vi "Instrument Mode.vi"(4 "SKIP(T)":bool, 6 "SET/GET":string(combo)="SET", 8 "error in":errorcluster {"code" format="%.0x"}, 9 "Select INST":string(combo)="INST SA", 11 "Session In":refnum<visa-resource-name>="TCPIP0::169.254.70.120::inst0::INSTR") -> (0 "error out":errorcluster={"status"=TRUE, "code"=-1073807339, "source"="VISA Write in Instrument Mode.vi"} {"code" format="%.0x"}, 2 "INST":string="INST SA", 3 "Session Out":refnum<visa-resource-name>="TCPIP0::169.254.70.120::inst0::INSTR")   [LabVIEW 2018]
doc: "Launches the Instrument I/O Assistant, which you can use to communicate with message-based instruments and graphically parse the response. For example you can communicate with an instrument that uses a serial, Ethernet, or GPIB interface."
panel:
  # ":INSTrument[:SELect] SA | RTSA | SEQAN | EMI | BASIC | WCDMA |\nEDGEGSM | WIMAXOFDMA | VSA | PNOISE | NFIGure | ADEMOD | BTooth |\nTDSCDMA | CDMA2K | CDMA1XEV | LTE | LTETDD | LTEAFDD | LTEATDD | MSR\n| DVB | DTMB | DCTV | ISDBT | CMMB | WLAN | CWLAN | CWIMAXOFDM |\nWIMAXFIXED | IDEN | RLC | SCPILC | VSA89601\n:INSTrument[:SELect]?"
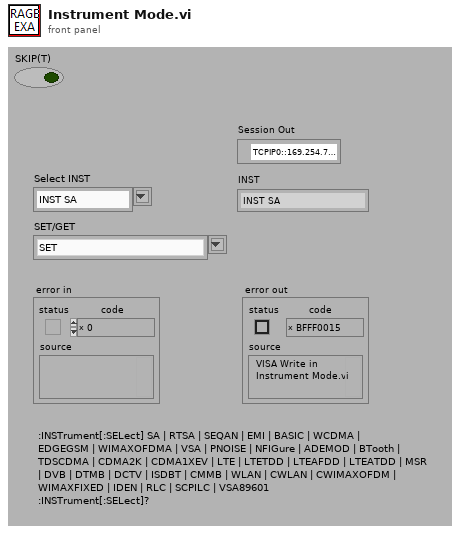
[diagram p1: front panel]
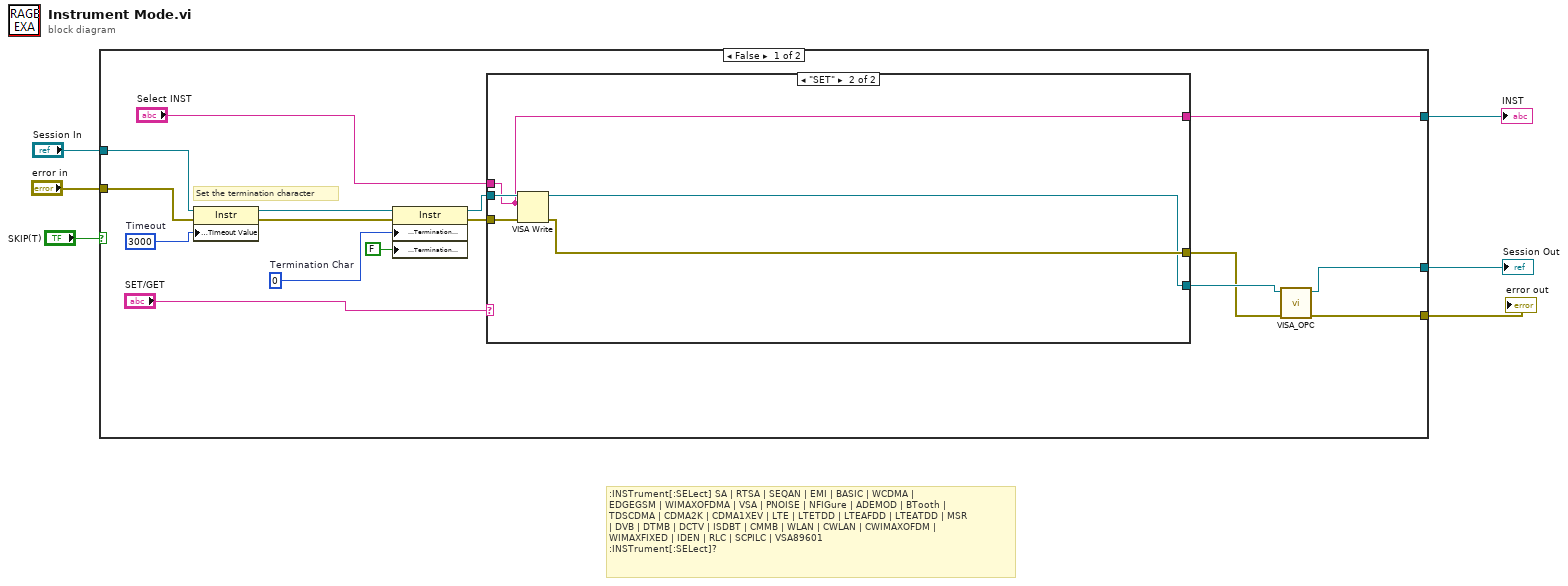
[diagram p0: block diagram]
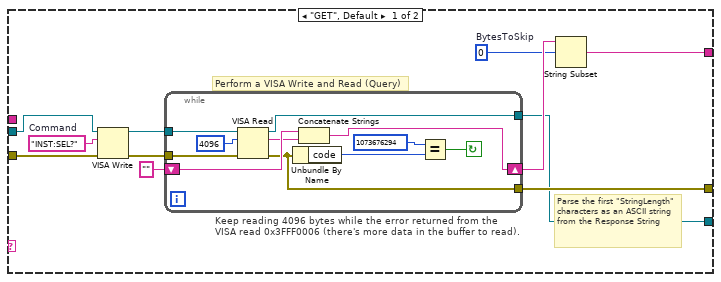
[diagram p2: hidden frame]
diagram:
  # ":INSTrument[:SELect] SA | RTSA | SEQAN | EMI | BASIC | WCDMA |\nEDGEGSM | WIMAXOFDMA | VSA | PNOISE | NFIGure | ADEMOD | BTooth |\nTDSCDMA | CDMA2K | CDMA1XEV | LTE | LTETDD | LTEAFDD | LTEATDD | MSR\n| DVB | DTMB | DCTV | ISDBT | CMMB | WLAN | CWLAN | CWIMAXOFDM |\nWIMAXFIXED | IDEN | RLC | SCPILC | VSA89601\n:INSTrument[:SELect]?"
  n1 = case shown="False" "SKIP(T)" {
    tunnel: "error in" -> [w21 w51]
    tunnel: "Session In" -> [w20 w50]
    tunnel: [w14 w50] -> w4
    tunnel: [w10 w50] -> w3
    tunnel: [w8 w51] -> w2
    frame False {
      w17 = u8 0  # Termination Char
      w22 = u32 3000  # Timeout
      # "Set the termination character"
      n2 = property class="Instr"(reference=w20, error in=w21, "General Settings:Timeout Value"=w22) -> (reference out=w16:refnum<visa-resource-name>, error out=w19:errorcluster)
      n3 = property class="Instr"(reference=w16, error in=w19, "Message Based Settings:Termination Character"=w17, "Message Based Settings:Termination Character Enable"=FALSE ("enable")) -> (reference out=w12:refnum<visa-resource-name>, error out=w18:errorcluster)
      n4 = case shown="\"SET\"" "SET/GET" {
        tunnel: w18 -> [w33 w49]
        tunnel: [w30 w48] -> w7
        tunnel: [w27 w45] -> w14
        tunnel: w12 -> [w24 w47]
        tunnel: "Select INST" -> [_ w45]
        tunnel: [w23 w46] -> w9
        frame "GET", Default {
          w25 = 0  # BytesToSkip
          w28 = "INST:SEL?"  # Command
          # "Parse the first \"StringLength\" characters as an ASCII string from the Response String"
          # "Perform a VISA Write and Read (Query)"
          # "Keep reading 4096 bytes while the error returned from the\nVISA read 0x3FFF0006 (there's more data in the buffer to read)."
          n5 = VISA Write(VISA resource name=w24, write buffer=w28, error in (no error)=w33) -> (VISA resource name out=w32:refnum<visa-resource-name>, error out=w31:errorcluster)  [unwired: 1 out]
          n6 = while {
            tunnel: w32 -> [w41]
            shift-right: [w35] -> w26
            shift-left: "" -> [w40]
            tunnel: w31 -> [w38]
            tunnel: [w37] -> w30
            tunnel: [w34] -> w23
            stop <- w36 continue-if-true
            n7 = VISA Read(VISA resource name=w41, byte count=u32 4096 ("byte count (0)"), error in (no error)=w38) -> (VISA resource name out=w34:refnum<visa-resource-name>, read buffer=w39:string, error out=w37:errorcluster)  [unwired: 1 out]
            n8 = Unbundle By Name(w37) -> ("code"=w43:i32)
            n9 = Concatenate Strings(w40, w39) -> (w35:string)
            n10 = Equal?(x=1073676294, y=w43) -> (x = y?=w36:bool)
          }
          n11 = String Subset(string=w26, offset (0)=w25) -> (substring=w27:string)  [unwired: 1 out]
        }
        frame "SET" {
          n12 = VISA Write(VISA resource name=w47, write buffer=w45, error in (no error)=w49) -> (VISA resource name out=w46:refnum<visa-resource-name>, error out=w48:errorcluster)  [unwired: 1 out]
        }
      }
      n13 = call "VISA_OPC.vi"("error in"=w7, "Session In"=w9) -> ("error out"=w8:errorcluster, "Session Out"=w10:refnum<visa-resource-name>)  [unwired: 7 in, 1 out]
    }
    frame True {
    }
  }
  "INST" <- w4
  "error out" <- w2
  "Session Out" <- w3
